vi "AtSpectrograph_acceptCommand_changeFilter.vi"(8 "error in (no error)":errorcluster, 11 "command_changeFilter_Ctl":T1) -> (0 "error out":errorcluster, 2 "function return":i32, 3 "command_changeFilter_Ctl out":T1)   [LabVIEW 2016, in "SALLV_AtSpectrograph.lvlib"]
doc: "int AtSpectrograph_shm_acceptCommand_changeFilterLV(AtSpectrograph_command_changeFilterLV *command_changeFilter_Ctl );"
uses:
  SALLV_AtSpectrograph.lvlib
  DataTypes/command_changeFilter.ctl
  SALLV_AtSpectrograph.so
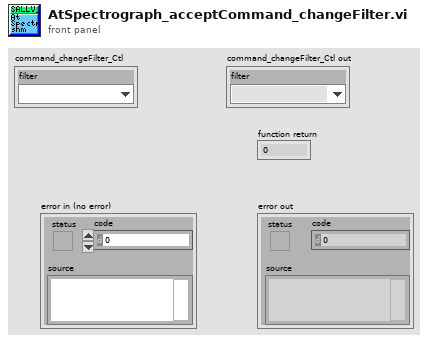
[diagram p1: front panel]
types:
  T1 = typedef "SALLV_AtSpectrograph.lvlib/command_changeFilter.ctl" = cluster{"filter":enum32{"", "slot0", "slot1", "slot2", "slot3"}}
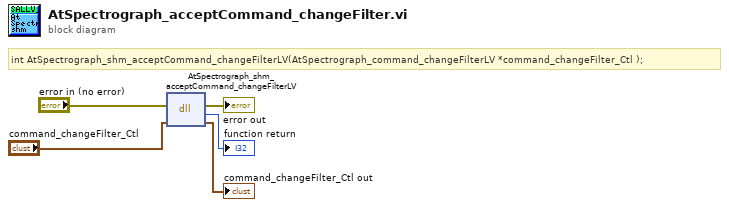
[diagram p0: block diagram]
diagram:
  # "int AtSpectrograph_shm_acceptCommand_changeFilterLV(AtSpectrograph_command_changeFilterLV *command_changeFilter_Ctl );"
  n1 = dll-call lib="home/harini/tcs/temp/SALLV_AtSpectrograph/SALLV_AtSpectrograph.*" fn="AtSpectrograph_shm_acceptCommand_changeFilterLV"(error in="error in (no error)", "command_changeFilter_Ctl"="command_changeFilter_Ctl") -> (error out=→"error out":errorcluster, →"function return":i32, "command_changeFilter_Ctl"=→"command_changeFilter_Ctl out":T1)  [unwired: 2 in, 1 out]
